vi "Initialize.vi"(8 "error in (no error)":errorcluster, 11 "UDP Transfer Rx User Interface in":refnum<class "UDP Transfer Rx User Interface.lvclass">) -> (0 "error out":errorcluster, 3 "UDP Transfer Rx User Interface out":refnum<class "UDP Transfer Rx User Interface.lvclass">)   [LabVIEW 2017, in "DSF Core.lvlib" / "UDP Transfer Rx User Interface.lvclass"]
uses:
  UDP Transfer Rx User Interface.lvclass
  C:/Git/DSF/Core/Classes/User Interface/User Interface.lvclass
  Configuration/Rx Transfer/UDP Transfer Rx Configuration.lvclass
  C:/Git/DSF/Core/Classes/Configuration/Configuration.lvclass
  User Interface.vi
  Classes/User Interface/User Interface.lvclass
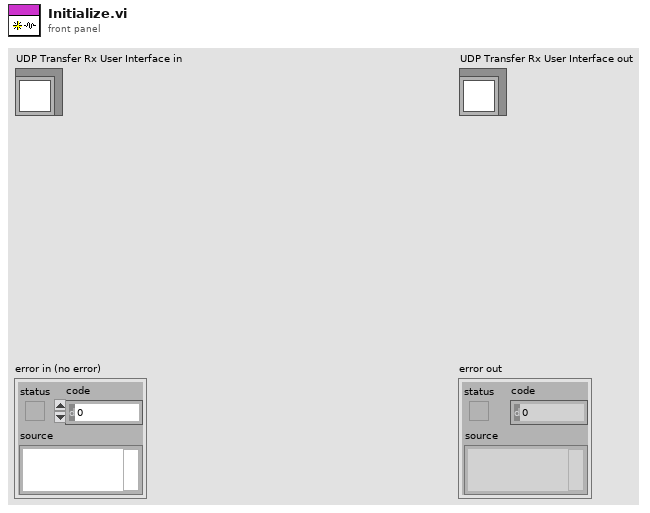
[diagram p1: front panel]
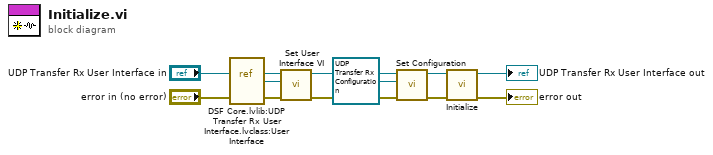
[diagram p0: block diagram]
diagram:
  n1 = vi-ref "DSF Core.lvlib:UDP Transfer Rx User Interface.lvclass:User Interface.vi"() -> (w1:refnum<vi>)
  n2 = call "Set User Interface VI.vi"("error in (no error)"="error in (no error)", "vi"=w1, "User Interface in"="UDP Transfer Rx User Interface in") -> ("error out"=w6:errorcluster, "User Interface out"=w3:refnum<class "UDP Transfer Rx User Interface.lvclass">)  [unwired: 7 in]
  n3 = call "Set Configuration.vi"("error in (no error)"=w6, "configuration"=refnum<class "UDP Transfer Rx Configuration.lvclass"> refnum ("DSF Core.lvlib:UDP Transfer Rx Configuration.lvclass"), "User Interface in"=w3) -> ("error out"=w5:errorcluster, "User Interface out"=w4:refnum<class "UDP Transfer Rx User Interface.lvclass">)  [unwired: 7 in]
  n4 = call-parent "Initialize.vi"("error in (no error)"=w5, "User Interface in"=w4) -> ("error out"=→"error out":errorcluster, "User Interface out"=→"UDP Transfer Rx User Interface out":refnum<class "UDP Transfer Rx User Interface.lvclass">)  [unwired: 8 in]
